vi "Get learning rates.vi"() -> (1 "Automatic LR":i32=-1, 4 "Continue? (T=yes)":bool=TRUE, 5 "Max LR":dbl=1.0 format="%.2f", 6 "Initial LR":dbl=5.0 format="%.2f", 7 "Min LR":dbl=0.005 format="%.2f")   [LabVIEW 2010]
panel:
  in  "Automatic LR after (iterations); -1 means off:":i32=-1
  in  "Initial LR":dbl=0.1 format="%.4f"
  in  "Minimum LR":dbl=0.005 format="%.4f"
  in  "Maximum LR":dbl=1.0 format="%.4f"
  in  "Exit":bool
  in  "OK":bool
  # "Set Learning Rate...\n(you can change any of these settings later)"
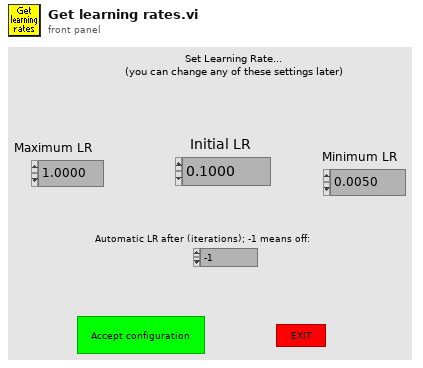
[diagram p1: front panel]
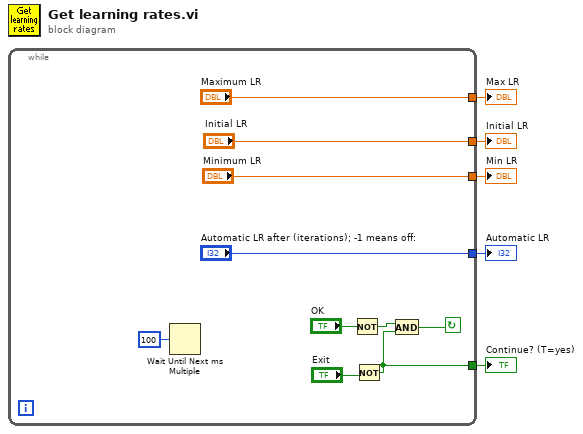
[diagram p0: block diagram]
diagram:
  n1 = while {
    tunnel: ["Automatic LR after (iterations); -1 means off:"] -> w1
    tunnel: ["Minimum LR"] -> w2
    tunnel: ["Initial LR"] -> w3
    tunnel: ["Maximum LR"] -> w4
    tunnel: [w11] -> w5
    stop <- w12 continue-if-true
    n2 = Wait Until Next ms Multiple(millisecond multiple=u32 100) -> ()  [unwired: 1 out]
    n3 = Not(x="OK") -> (.not. x?=w14:bool)
    n4 = Not(x="Exit") -> (.not. x?=w11:bool)
    n5 = And(x=w14, y=w11) -> (x .and. y?=w12:bool)
  }
  "Continue? (T=yes)" <- w5
  "Max LR" <- w4
  "Initial LR" <- w3
  "Min LR" <- w2
  "Automatic LR" <- w1
